vi "ADCS.TesterPresent.vi"(7 "Enabled?":bool, 8 "error in (no error)":errorcluster, 10 "Reset":bool, 11 "State Variables in":T1={"TCP Refs"={"Connection List"=refnum, "listener ID"=refnum}, "Parameters"={"Properties"={"Name"="", "CAN"={"CAN Interface"=enum."CAN0", "Baud Rate"=0, "Diagnostic Protocol"=enum."GMLAN", "Transport Protocol"=enum."ISO TP - Normal Mode", "Transmit ID"=0, "Receive ID"=0, "Transmit Extension"=0, "Receive Extension"=0, "Receive UUDT ID"=0, "Enable Stream"=FALSE, "VW TP Channel ID"=0, "Security"={"Source DLL Path"=path "", "Security Level"=0, "Target DLL Path"=path ""}, "Fill Frame"=FALSE, "Fill Byte"=255, "Termination"=FALSE}, "986x"={"Enable"=FALSE, "RIO Device"=0, "Bitfile"=path ""}, "Reads"=[], "Frames Lookup"=variant, "Writes"=[], "DPIDs"=[], "DPID Lookup"=variant, "DTC descriptor"={"DTC Byte Length"=0, "Status Byte Length"=0, "Add Data Byte Length"=0, "Byte Order"=enum."Motorola"}, "Created DTCs"=0}, "ChanRefs"={"ToVS.Reads"={"Name"="", "Write to VS Engine FIFO"=refnum, "Pairs"={"Refs"=[], "Values"=[]}}, "ToVS.DTCs"={"Name"="", "Write to VS Engine FIFO"=refnum, "Pairs"={"Refs"=[], "Values"=[]}}, "ToVS.DTCCount"={"Name"="", "Write to VS Engine FIFO"=refnum, "Pairs"={"Refs"=[], "Values"=[]}}, "ToVS.Status"={"Name"="", "Write to VS Engine FIFO"=refnum, "Pairs"={"Refs"=[], "Values"=[]}}, "FromVS.Writes"={"Name"="", "Read from VS Engine FIFO"=refnum, "Pairs"={"Refs"=[], "Values"=[]}}, "Cmds"={"Name"="", "Write to VS Engine FIFO"=refnum, "Read from VS Engine FIFO"=refnum, "Pairs"={"Chan Refs"=[], "Prev. Values"=[]}}, "Triggers"={"Name"="", "Write to VS Engine FIFO"=refnum, "Read from VS Engine FIFO"=refnum, "Pairs"={"Chan Refs"=[], "Prev. Values"=[]}}}}, "ADCS Connection"={"Diag CAN Handle"=0, "Transport Protocol"=enum."ISO TP - Normal Mode", "Receive Address Extension"=0, "Transmit Address Extension"=0, "Receive CAN Id"=0, "Transmit CAN Id"=0, "Diag CAN Queue"=refnum, "Log Frames ?"=FALSE, "My TP Address"=0, "Other TP Address"=0, "T1"=0, "T2"=0, "T3"=0, "T4"=0, "Tx SN"=0, "Block Size"=0, "Rx SN"=0, "VW TP Initialized?"=FALSE, "Tx block no"=0, "baud rate"=0, "Interface"="", "Channel Diag CAN Handle"=0, "UDP Connection ID"=refnum, "TCP Connection ID"=refnum, "Target IP Addr"=0, "Source Address"=0, "Target Address"=0, "Send Header NACK?"=FALSE, "DLL Handle"=0, "NAD"=0, "Time Stamp read first"=0.0, "Time Stamp read last"=0.0, "Time Stamp write first"=0.0, "Time Stamp write last"=0.0, "Time Stamp write"=0.0, "Time Stamp read"=0.0}, "XNET References"={"Database"="", "GMLAN DPID Session"="", "Cluster"=""}, "BufferedCmds"=refnum, "XNETEngine (GMLAN)"=refnum, "Process"=refnum} {"Parameters"."ChanRefs"."Triggers"."Pairs"."Chan Refs" format="%.0x"; "Parameters"."ChanRefs"."Cmds"."Pairs"."Chan Refs" format="%.0x"; "Parameters"."ChanRefs"."ToVS.Status"."Pairs"."Refs" format="%.0x"; "Parameters"."ChanRefs"."ToVS.DTCCount"."Pairs"."Refs" format="%.0x"; "Parameters"."ChanRefs"."ToVS.DTCs"."Pairs"."Refs" format="%.0x"; "Parameters"."ChanRefs"."ToVS.Reads"."Pairs"."Refs" format="%.0x"; "Parameters"."Properties"."Writes"."Signals"."Byte Order" items=["Little Endian", "Big Endian"]; "Parameters"."Properties"."Writes"."Signals"."Data Type" items=["Signed", "Unsigned", "IEEE Float"]; "Parameters"."Properties"."CAN"."Fill Byte" format="%.0x"; "Parameters"."Properties"."CAN"."VW TP Channel ID" format="%.0x"; "Parameters"."Properties"."CAN"."Receive UUDT ID" format="%.0x"; "Parameters"."Properties"."CAN"."Receive Extension" format="%.0x"; "Parameters"."Properties"."CAN"."Transmit Extension" format="%.0x"; "Parameters"."Properties"."CAN"."Receive ID" format="%.0x"; "Parameters"."Properties"."CAN"."Transmit ID" format="%.0x"; "Parameters"."Properties"."Reads"."Signals"."Byte Order" items=["Little Endian", "Big Endian"]; "Parameters"."Properties"."Reads"."Signals"."Data Type" items=["Signed", "Unsigned", "IEEE Float"]}) -> (0 "error out":errorcluster, 3 "State Variables out":T1={"TCP Refs"={"Connection List"=refnum, "listener ID"=refnum}, "Parameters"={"Properties"={"Name"="", "CAN"={"CAN Interface"=enum."CAN0", "Baud Rate"=0, "Diagnostic Protocol"=enum."GMLAN", "Transport Protocol"=enum."ISO TP - Normal Mode", "Transmit ID"=0, "Receive ID"=0, "Transmit Extension"=0, "Receive Extension"=0, "Receive UUDT ID"=0, "Enable Stream"=FALSE, "VW TP Channel ID"=0, "Security"={"Source DLL Path"=path "", "Security Level"=0, "Target DLL Path"=path ""}, "Fill Frame"=FALSE, "Fill Byte"=255, "Termination"=FALSE}, "986x"={"Enable"=FALSE, "RIO Device"=0, "Bitfile"=path ""}, "Reads"=[], "Frames Lookup"=variant, "Writes"=[], "DPIDs"=[], "DPID Lookup"=variant, "DTC descriptor"={"DTC Byte Length"=0, "Status Byte Length"=0, "Add Data Byte Length"=0, "Byte Order"=enum."Motorola"}, "Created DTCs"=0}, "ChanRefs"={"ToVS.Reads"={"Name"="", "Write to VS Engine FIFO"=refnum, "Pairs"={"Refs"=[], "Values"=[]}}, "ToVS.DTCs"={"Name"="", "Write to VS Engine FIFO"=refnum, "Pairs"={"Refs"=[], "Values"=[]}}, "ToVS.DTCCount"={"Name"="", "Write to VS Engine FIFO"=refnum, "Pairs"={"Refs"=[], "Values"=[]}}, "ToVS.Status"={"Name"="", "Write to VS Engine FIFO"=refnum, "Pairs"={"Refs"=[], "Values"=[]}}, "FromVS.Writes"={"Name"="", "Read from VS Engine FIFO"=refnum, "Pairs"={"Refs"=[], "Values"=[]}}, "Cmds"={"Name"="", "Write to VS Engine FIFO"=refnum, "Read from VS Engine FIFO"=refnum, "Pairs"={"Chan Refs"=[], "Prev. Values"=[]}}, "Triggers"={"Name"="", "Write to VS Engine FIFO"=refnum, "Read from VS Engine FIFO"=refnum, "Pairs"={"Chan Refs"=[], "Prev. Values"=[]}}}}, "ADCS Connection"={"Diag CAN Handle"=0, "Transport Protocol"=enum."ISO TP - Normal Mode", "Receive Address Extension"=0, "Transmit Address Extension"=0, "Receive CAN Id"=0, "Transmit CAN Id"=0, "Diag CAN Queue"=refnum, "Log Frames ?"=FALSE, "My TP Address"=0, "Other TP Address"=0, "T1"=0, "T2"=0, "T3"=0, "T4"=0, "Tx SN"=0, "Block Size"=0, "Rx SN"=0, "VW TP Initialized?"=FALSE, "Tx block no"=0, "baud rate"=0, "Interface"="", "Channel Diag CAN Handle"=0, "UDP Connection ID"=refnum, "TCP Connection ID"=refnum, "Target IP Addr"=0, "Source Address"=0, "Target Address"=0, "Send Header NACK?"=FALSE, "DLL Handle"=0, "NAD"=0, "Time Stamp read first"=0.0, "Time Stamp read last"=0.0, "Time Stamp write first"=0.0, "Time Stamp write last"=0.0, "Time Stamp write"=0.0, "Time Stamp read"=0.0}, "XNET References"={"Database"="", "GMLAN DPID Session"="", "Cluster"=""}, "BufferedCmds"=refnum, "XNETEngine (GMLAN)"=refnum, "Process"=refnum} {"Parameters"."ChanRefs"."Triggers"."Pairs"."Chan Refs" format="%.0x"; "Parameters"."ChanRefs"."Cmds"."Pairs"."Chan Refs" format="%.0x"; "Parameters"."ChanRefs"."ToVS.Status"."Pairs"."Refs" format="%.0x"; "Parameters"."ChanRefs"."ToVS.DTCCount"."Pairs"."Refs" format="%.0x"; "Parameters"."ChanRefs"."ToVS.DTCs"."Pairs"."Refs" format="%.0x"; "Parameters"."ChanRefs"."ToVS.Reads"."Pairs"."Refs" format="%.0x"; "Parameters"."Properties"."Writes"."Signals"."Byte Order" items=["Little Endian", "Big Endian"]; "Parameters"."Properties"."Writes"."Signals"."Data Type" items=["Signed", "Unsigned", "IEEE Float"]; "Parameters"."Properties"."CAN"."Fill Byte" format="%.0x"; "Parameters"."Properties"."CAN"."VW TP Channel ID" format="%.0x"; "Parameters"."Properties"."CAN"."Receive UUDT ID" format="%.0x"; "Parameters"."Properties"."CAN"."Receive Extension" format="%.0x"; "Parameters"."Properties"."CAN"."Transmit Extension" format="%.0x"; "Parameters"."Properties"."CAN"."Receive ID" format="%.0x"; "Parameters"."Properties"."CAN"."Transmit ID" format="%.0x"; "Parameters"."Properties"."Reads"."Signals"."Byte Order" items=["Little Endian", "Big Endian"]; "Parameters"."Properties"."Reads"."Signals"."Data Type" items=["Signed", "Unsigned", "IEEE Float"]})   [LabVIEW 2015, in "Diagnostics Addon Engine.lvlib"]
uses:
  Diagnostics Addon Engine.lvlib
  Types/Diagnostics.State.ctl
  <vilib>/NI/NI VeriStand Inline Async API/_VS Inline Async API/Process/Process.lvclass
  Types/TCP.Refs.ctl
  STM/STM Lookup Table Ref.ctl
  Types/Engine.State.ctl
  Shared/Types/SysDef.Compile.Properties.ctl
  Shared/Types/CAN.ctl
  Shared/Types/CAN.Interface.ctl
  Shared/Types/Protocol.ctl
  Shared/Types/Transport.ctl
  Shared/Types/Security.ctl
  Shared/Types/986x.ctl
  Shared/Types/Frame.Compile.ctl
  Shared/Types/Type.ctl
  Shared/Types/Signal.ctl
  Shared/Types/DPID.ctl
  Shared/Types/DPID.Rate.ctl
  Shared/Types/DTCDescriptor.ctl
  Types/Engine.Refs.ctl
  Inline Async API/Controls/Write To VS Engine.ctl
  <vilib>/NI Veristand/Custom Device API/Data Reference.ctl
  Inline Async API/Controls/Read From VS Engine.ctl
  <vilib>/NI Veristand/Custom Device API/Block Data Reference.ctl
  Inline Async API/Controls/ReadWrite Data.ctl
  <vilib>/Automotive Diagnostic Command Set/Diagnostic Transport.llb/Diag Reference.ctl
  <vilib>/Automotive Diagnostic Command Set/Diagnostic Transport.llb/Transport Protocol Selector.ctl
  <vilib>/Automotive Diagnostic Command Set/Diagnostic Transport.llb/Diag CAN Frame Log.ctl
  Types/XNET.Refs.ctl
  <vilib>/NI/AMC/Message Queue.ctl
  <vilib>/NI/AMC/Message.ctl
  <vilib>/NI/Tools/Keyed Array/KeyedArray.ctl
  GMLAN/_SubVIs/TesterPresent_Parameter.ctl
  GMLAN/Utilities/GMLAN Service Broadcast.vi
  <vilib>/Automotive Diagnostic Command Set/Diagnostic Transport.llb/Apply Success Failure Error.vi
  <vilib>/Automotive Diagnostic Command Set/Diagnostic Transport.llb/Diagnostic Service.vi
  <vilib>/Automotive Diagnostic Command Set/Diagnostic Transport.llb/Apply Diagnostic Error.vi
  <vilib>/Automotive Diagnostic Command Set/Diagnostic Transport.llb/Diagnostic Response Recv.vi
  <vilib>/Automotive Diagnostic Command Set/Diagnostic Transport.llb/Diagnostic Service Send.vi
  <vilib>/Automotive Diagnostic Command Set/Diagnostic Transport.llb/Diag Globals.vi
  GMLAN/GMLAN.lvlib
  Shared/Diagnostics Addon Shared.lvlib
  <vilib>/NI Veristand/Custom Device API/Custom Device API.lvlib
  Inline Async API/Inline Async API.lvlib
  <vilib>/addons/Automotive Diagnostic Command Set/NI_Automotive Diagnostic Command Set.lvlib
  <vilib>/NI/Tools/Keyed Array/Tools_KeyedArray.lvlib
  <vilib>/NI/AMC/AMC.lvlib
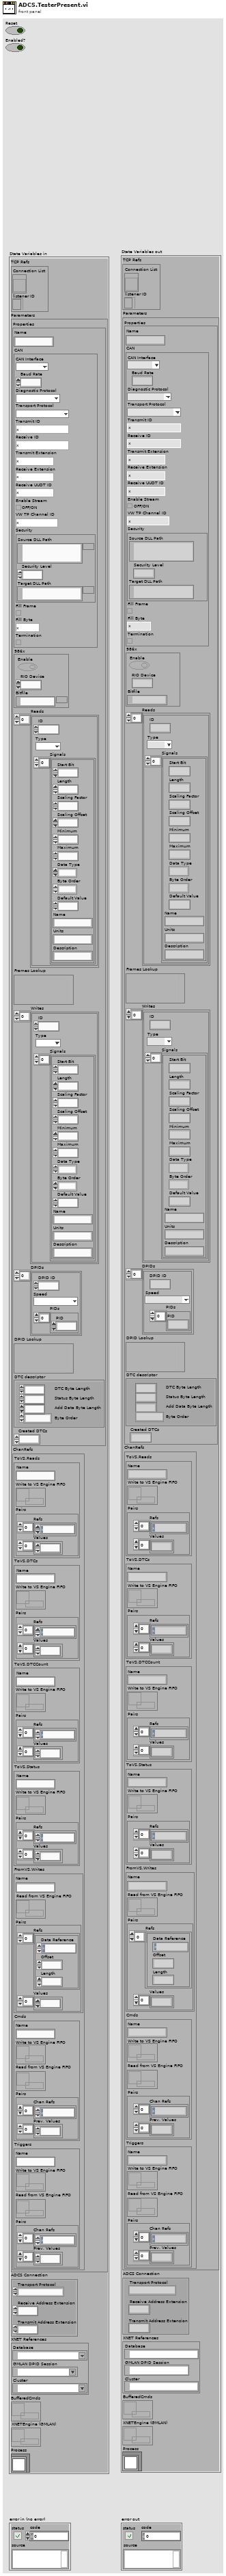
[diagram p1: front panel]
types:
  T1 = typedef "Diagnostics Addon Engine.lvlib/Diagnostics.State.ctl" = cluster{"TCP Refs":T2, "Parameters":T4, "ADCS Connection":T24, "XNET References":T26, "BufferedCmds":T27, "XNETEngine (GMLAN)":T27, "Process":refnum<class "Process.lvclass">}
  T2 = typedef "Diagnostics Addon Engine.lvlib/TCP.Refs.ctl" = cluster{"Connection List":T3, "listener ID":refnum<k5>}
  T3 = typedef "Diagnostics Addon Engine.lvlib/STM Lookup Table Ref.ctl" = refnum<vi>
  T4 = typedef "Diagnostics Addon Engine.lvlib/Engine.State.ctl" = cluster{"Properties":T5, "ChanRefs":T18}
  T5 = typedef "Diagnostics Addon Shared.lvlib/SysDef.Compile.Properties.ctl" = cluster{"Name":string, "CAN":T6, "986x":T11, "Reads":T12[], "Frames Lookup":variant, "Writes":T12[], "DPIDs":T15[], "DPID Lookup":variant, "DTC descriptor":T17, "Created DTCs":u32}
  T6 = typedef "Diagnostics Addon Shared.lvlib/CAN.ctl" = cluster{"CAN Interface":T7, "Baud Rate":u32, "Diagnostic Protocol":T8, "Transport Protocol":T9, "Transmit ID":u32, "Receive ID":u32, "Transmit Extension":u8, "Receive Extension":u8, "Receive UUDT ID":u32, "Enable Stream":bool, "VW TP Channel ID":u32, "Security":T10, "Fill Frame":bool, "Fill Byte":u8, "Termination":bool}
  T7 = typedef "Diagnostics Addon Shared.lvlib/CAN.Interface.ctl" = enum16{"CAN0", "CAN1", "CAN2", "CAN3", "CAN4", "CAN5", "CAN6", "CAN7", "CAN8", "CAN9", "CAN10", "CAN11", "CAN12", "CAN13", "CAN14", "CAN15", "CAN16", "CAN17", "CAN18", "CAN19", "CAN20", "CAN21", "CAN22", "CAN23", "CAN24", "CAN25", "CAN26", "CAN27", "CAN28", "CAN29", "CAN30", "CAN31", "CAN32", "CAN33", "CAN34", "CAN35", "CAN36", "CAN37", "CAN38", "CAN39", "CAN40", "CAN41", "CAN42", "CAN43", "CAN44", "CAN45", "CAN46", "CAN47", "CAN48", "CAN49", "CAN50", "CAN51", "CAN52", "CAN53", "CAN54", "CAN55", "CAN56", "CAN57", "CAN58", "CAN59", "CAN60", "CAN61", "CAN62", "CAN63", "CAN 256 (Virtual)", "CAN 257 (Virtual)"}
  T8 = typedef "Diagnostics Addon Shared.lvlib/Protocol.ctl" = enum16{"GMLAN", "KWP-2000", "UDS", "User-Defined"}
  T9 = typedef "Diagnostics Addon Shared.lvlib/Transport.ctl" = enum16{"ISO TP - Normal Mode", "ISO TP - Mixed Mode", "VW TP 2.0", "Diagnostics on IP"}
  T10 = typedef "Diagnostics Addon Shared.lvlib/Security.ctl" = cluster{"Source DLL Path":path, "Security Level":u8, "Target DLL Path":path}
  T11 = typedef "Diagnostics Addon Shared.lvlib/986x.ctl" = cluster{"Enable":bool, "RIO Device":u16, "Bitfile":path}
  T12 = typedef "Diagnostics Addon Shared.lvlib/Frame.Compile.ctl" = cluster{"ID":u32, "Type":T13, "Signals":T14[]}
  T13 = typedef "Diagnostics Addon Shared.lvlib/Type.ctl" = enum16{"DID", "CDID", "PID", "CPID", "Read Memory", "Write Memory", "DTC Control", "IO Cmd", "IO Resp", "Routine Start Cmd", "Routine Start Resp", "Routine Request Cmd", "Routine Request Resp", "Routine Stop Cmd", "Routine Stop Resp", "UserDefined Cmd", "UserDefined Rsp"}
  T14 = typedef "Diagnostics Addon Shared.lvlib/Signal.ctl" = cluster{"Start Bit":u32, "Length":u32, "Scaling Factor":dbl, "Scaling Offset":dbl, "Minimum":dbl, "Maximum":dbl, "Data Type":u32, "Byte Order":u32, "Default Value":dbl, "Name":string, "Units":string, "Description":string}
  T15 = typedef "Diagnostics Addon Shared.lvlib/DPID.ctl" = cluster{"DPID ID":u8, "Speed":T16, "PIDs":u16[]}
  T16 = typedef "Diagnostics Addon Shared.lvlib/DPID.Rate.ctl" = enum16{"Slow", "Medium", "Fast"}
  T17 = typedef "Diagnostics Addon Shared.lvlib/DTCDescriptor.ctl" = cluster{"DTC Byte Length":i32, "Status Byte Length":i32, "Add Data Byte Length":i32, "Byte Order":enum16{"Motorola", "Intel"}}
  T18 = typedef "Diagnostics Addon Engine.lvlib/Engine.Refs.ctl" = cluster{"ToVS.Reads":T19, "ToVS.DTCs":T19, "ToVS.DTCCount":T19, "ToVS.Status":T19, "FromVS.Writes":T21, "Cmds":T23, "Triggers":T23}
  T19 = typedef "Diagnostics Addon Engine.lvlib/Inline Async API.lvlib/Write To VS Engine.ctl" = cluster{"Name":string, "Write to VS Engine FIFO":refnum<k33>, "Pairs":cluster{"Refs":T20[], "Values":dbl[]}}
  T20 = typedef "Custom Device API.lvlib/Data Reference.ctl" = i32
  T21 = typedef "Diagnostics Addon Engine.lvlib/Inline Async API.lvlib/Read From VS Engine.ctl" = cluster{"Name":string, "Read from VS Engine FIFO":refnum<k33>, "Pairs":cluster{"Refs":T22[], "Values":dbl[]}}
  T22 = typedef "Custom Device API.lvlib/Block Data Reference.ctl" = cluster{"Data Reference":T20, "Offset":u64, "Length":u64}
  T23 = typedef "Diagnostics Addon Engine.lvlib/Inline Async API.lvlib/ReadWrite Data.ctl" = cluster{"Name":string, "Write to VS Engine FIFO":refnum<k33>, "Read from VS Engine FIFO":refnum<k33>, "Pairs":cluster{"Chan Refs":T20[], "Prev. Values":dbl[]}}
  T24 = typedef "NI_Automotive Diagnostic Command Set.lvlib/Diag Reference.ctl" = cluster{"Diag CAN Handle":u32, "Transport Protocol":T25, "Receive Address Extension":u8, "Transmit Address Extension":u8, "Receive CAN Id":u32, "Transmit CAN Id":u32, "Diag CAN Queue":refnum<queue>, "Log Frames ?":bool, "My TP Address":u8, "Other TP Address":u8, "T1":u16, "T2":u16, "T3":u16, "T4":u16, "Tx SN":u8, "Block Size":u8, "Rx SN":u8, "VW TP Initialized?":bool, "Tx block no":u8, "baud rate":u32, "Interface":string, "Channel Diag CAN Handle":u32, "UDP Connection ID":refnum<k16>, "TCP Connection ID":refnum<k5>, "Target IP Addr":u32, "Source Address":u16, "Target Address":u16, "Send Header NACK?":bool, "DLL Handle":u32, "NAD":u8, "Time Stamp read first":dbl, "Time Stamp read last":dbl, "Time Stamp write first":dbl, "Time Stamp write last":dbl, "Time Stamp write":dbl, "Time Stamp read":dbl}
  T25 = typedef "NI_Automotive Diagnostic Command Set.lvlib/Transport Protocol Selector.ctl" = enum16{"ISO TP - Normal Mode", "ISO TP - Mixed Mode", "VW TP 2.0", "Diagnostics on IP", "ISO TP LIN"}
  T26 = typedef "Diagnostics Addon Engine.lvlib/XNET.Refs.ctl" = cluster{"Database":refnum<k21>, "GMLAN DPID Session":refnum<k21>, "Cluster":refnum<k21>}
  T27 = typedef "AMC.lvlib/Message Queue.ctl" = refnum<queue>
  T28 = typedef "GMLAN.lvlib/TesterPresent_Parameter.ctl" = enum8{"SpecificECU", "EntireNetwork"}
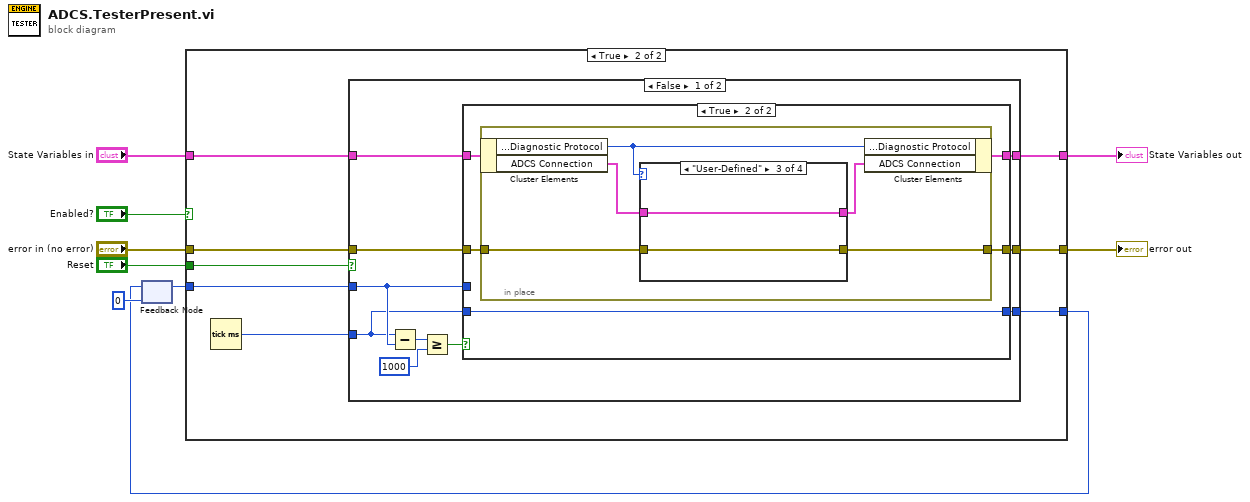
[diagram p0: block diagram]
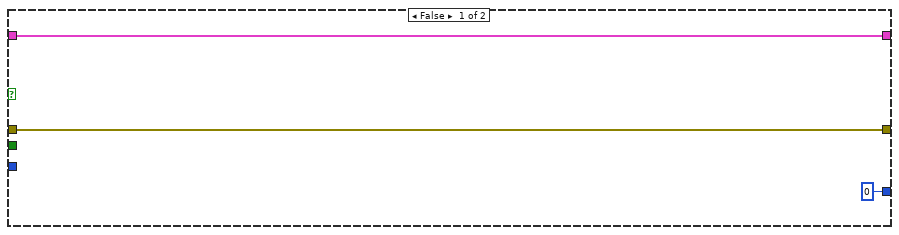
[diagram p2: hidden frame]
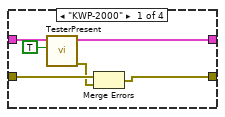
[diagram p4: hidden frame]
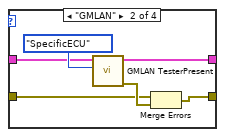
[diagram p5: hidden frame]
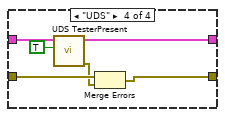
[diagram p6: hidden frame]
diagram:
  n1 = feedback #1(u32 0 ("millisecond timer value")) -> (w1:u32)
  n2 = case shown="True" "Enabled?" {
    tunnel: "error in (no error)" -> [w12 w20]
    tunnel: [w11 w19] -> w8
    tunnel: "State Variables in" -> [w11 w18]
    tunnel: [w12 w17] -> w6
    tunnel: "Reset" -> [_ w15]
    tunnel: [u32 0 ("millisecond timer value") w14] -> w2
    tunnel: w1 -> [_ w13]
    frame False {
    }
    frame True {
      n3 = Tick Count (ms)() -> (millisecond timer value=w16:u32)
      n4 = case shown="False" w15 {
        tunnel: w20 -> [w30 w65]
        tunnel: [w29 w64] -> w19
        tunnel: w18 -> [w28 w64]
        tunnel: [w27 w65] -> w17
        tunnel: w13 -> [w26 _]
        tunnel: w16 -> [w25 w66]
        tunnel: [w24 w66] -> w14
        frame False {
          n5 = Subtract(x=w25, y=w26) -> (x-y=w21:u32)
          n6 = Greater Or Equal?(x=w21, y=u32 1000) -> (x >= y?=w23:bool)
          n7 = case shown="True" w23 {
            tunnel: w30 -> [w32 w37]
            tunnel: [w33 w38] -> w24
            tunnel: w26 -> [w33 _]
            tunnel: w25 -> [_ w38]
            tunnel: [w32 w36] -> w27
            tunnel: w28 -> [w31 w35]
            tunnel: [w31 w34] -> w29
            frame False {
            }
            frame True {
              # "send tester present"
              n8 = in-place {
                in-place-border: w37 -> [w43]
                in-place-border: [w42] -> w36
                n9 = in-place-cluster #2(w35) -> ("Parameters.Properties.CAN.Diagnostic Protocol"=w39:T8, "ADCS Connection"=w41:T24)
                n10 = case shown="\"User-Defined\"" w39 {
                  tunnel: w43 -> [w46 w51 w56 w63]
                  tunnel: [w44 w50 w56 w61] -> w42
                  tunnel: w41 -> [w49 w54 w57 w59]
                  tunnel: [w48 w53 w57 w58] -> w40
                  frame "KWP-2000" {
                    n11 = call <vilib>:"TesterPresent.vi"("response required?"=TRUE, "diag ref in"=w49) -> ("error out"=w45:errorcluster, "diag ref out"=w48:T24)  [unwired: 7 in, 1 out]
                    n12 = Merge Errors(w46, w45) -> (w44:errorcluster)
                  }
                  frame "GMLAN" {
                    n13 = call "GMLAN TesterPresent.vi"("Parameter"=TesterPresent_Parameter."SpecificECU", "diag ref in"=w54) -> ("error out"=w52:errorcluster, "diag ref out"=w53:T24)  [unwired: 7 in, 1 out]
                    n14 = Merge Errors(w51, w52) -> (w50:errorcluster)
                  }
                  frame "User-Defined" {
                  }
                  frame "UDS" {
                    n15 = call <vilib>:"UDS TesterPresent.vi"("response required?"=TRUE, "diag ref in"=w59) -> ("error out"=w62:errorcluster, "diag ref out"=w58:T24)  [unwired: 7 in, 1 out]
                    n16 = Merge Errors(w63, w62) -> (w61:errorcluster)
                  }
                }
                n17 = in-place-cluster #2("Parameters.Properties.CAN.Diagnostic Protocol"=w39, "ADCS Connection"=w40) -> (w34:T1)
              }
            }
          }
        }
        frame True {
        }
      }
    }
  }
  "State Variables out" <- w8
  "error out" <- w6
  n18 = feedback-in #1(w2) -> ()
